vi "MDF4 Add Channel.vi"(6 "Channel ID":u64, 7 "Channel Name":string, 8 "Error In":errorcluster, 9 "Channel Group Reference in":i64, 10 "Data Group Reference in":i64, 11 "MDF4 File Reference in":i64) -> (0 "Error Out":errorcluster, 2 "Data Group Reference out":i64, 3 "MDF4 File Reference out":i64)   [LabVIEW 2019, in "MD4Logger Engine.lvlib"]
uses:
  MD4Logger Engine.lvlib
  <vilib>/Utility/error.llb/Error Cluster From Error Code.vi
  <vilib>/ErrorRing/Error Ring.xnode
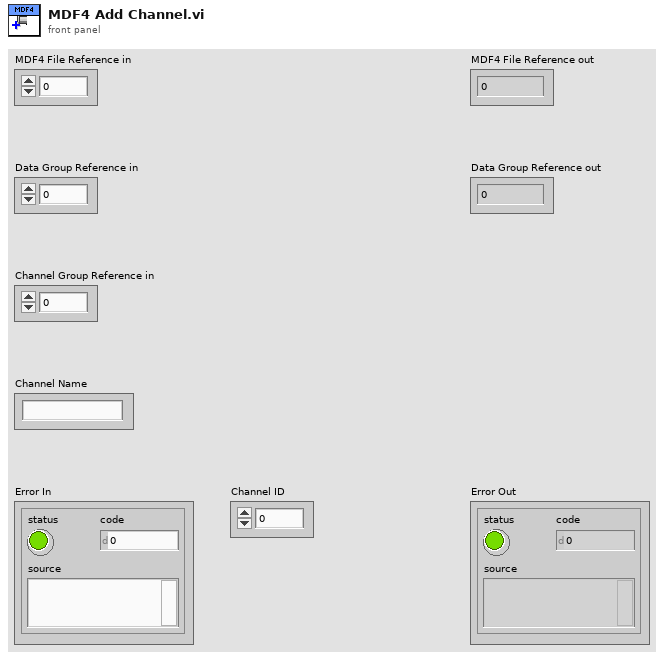
[diagram p1: front panel]
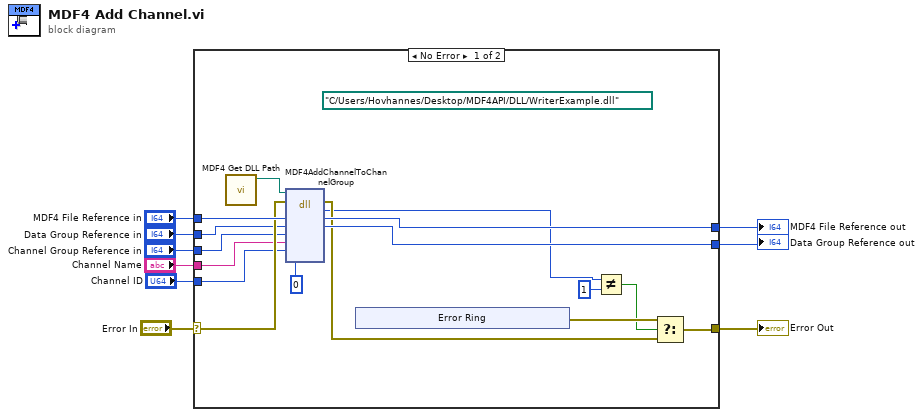
[diagram p0: block diagram]
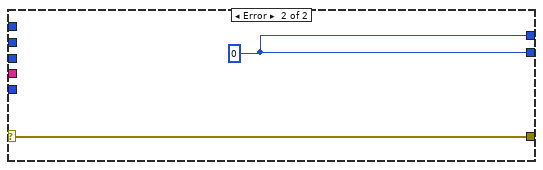
[diagram p2: hidden frame]
diagram:
  n1 = case shown="No Error" "Error In" {
    selector: "Error In" -> [w24 w32]
    tunnel: "MDF4 File Reference in" -> [w25 _]
    tunnel: [w19 w32] -> w7
    tunnel: [w23 w31] -> w6
    tunnel: [w22 w31] -> w5
    tunnel: "Data Group Reference in" -> [w21 _]
    tunnel: "Channel Group Reference in" -> [w17 _]
    tunnel: "Channel Name" -> [w16 _]
    tunnel: "Channel ID" -> [w15 _]
    frame No Error {
      (unwired) path "C:/Users/Hovhannes/Desktop/MDF4API/DLL/WriterExample.dll" ("path in")
      n2 = call "MDF4 Get DLL Path.vi"() -> ("DLL Path Out"=w10:path)  [unwired: 11 in]
      n3 = dll-call lib="C:/Users/Hovhannes/Desktop/MDF4API/DLL/WriterExample.dll" fn="MDF4AddChannelToChannelGroup"(path in=w10, error in=w24, "m4"=w25, "dg"=w21, "cg"=w17, "channel_name"=w16, "id"=w15, "cn"=i64 0) -> (error out=w18:errorcluster, "return type"=w13:i32, "m4"=w22:i64, "dg"=w23:i64)  [unwired: 5 in, 1 out]
      n4 = xnode "Error Ring"() -> ("error out"=w20:errorcluster)
      n5 = Not Equal?(x=w13, y=1) -> (x != y?=w12:bool)
      n6 = Select(t=w20, s=w12, f=w18) -> (s? t:f=w19:errorcluster)
    }
    frame Error {
      w31 = i64 0 ("m4")
    }
  }
  "Data Group Reference out" <- w6
  "Error Out" <- w7
  "MDF4 File Reference out" <- w5
